vi "handle name deletion.vi"(2 "error in (no error)":errorcluster, 3 "String":string, 4 "VISA resource name":refnum<visa-resource-name>) -> (0 "error out":errorcluster, 1 "VISA resource name out":refnum<visa-resource-name>)   [LabVIEW 2018]
uses:
  <instrlib>/Tektronix AWG 5000 7000 Series/Tektronix AWG 5000 7000 Series.lvlib
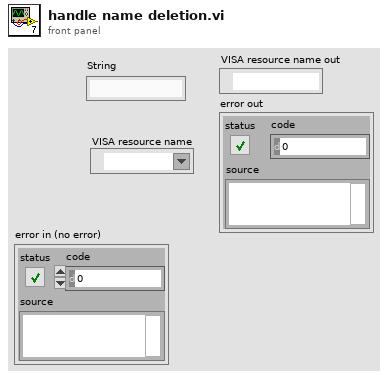
[diagram p1: front panel]
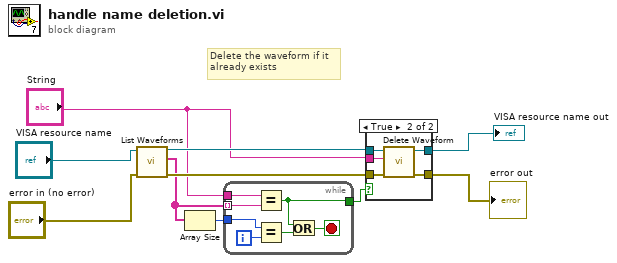
[diagram p0: block diagram]
diagram:
  # "Delete the waveform if it\nalready exists"
  n1 = call <instrlib>:"List Waveforms.vi"("error in (no error)"="error in (no error)", "VISA resource name"="VISA resource name") -> ("error out"=w9:errorcluster, "Waveform List"=w6:string[], "VISA resource name out"=w10:refnum<visa-resource-name>)  [unwired: 7 in]
  n2 = Array Size(array=w6) -> (size(s)=w7:i32)
  n3 = while {
    tunnel: [w15] -> w8
    tunnel: w7 -> [w13]
    tunnel: "String" -> [w12]
    tunnel: w6 -> [w11] mode=indexing
    i -> [w17]
    stop <- w14 stop-if-true
    n4 = Equal?(x=w12, y=w11) -> (x = y?=w15:bool)
    n5 = Equal?(x=w13, y=w17) -> (x = y?=w16:bool)
    n6 = Or(x=w15, y=w16) -> (x .or. y?=w14:bool)
  }
  n7 = case shown="True" w8 {
    tunnel: w10 -> [w19 w24]
    tunnel: [w19 w23] -> w4
    tunnel: w9 -> [w18 w22]
    tunnel: [w18 w21] -> w3
    tunnel: "String" -> [_ w20]
    frame False {
    }
    frame True {
      n8 = call <instrlib>:"Delete Waveform.vi"("error in (no error)"=w22, "Waveform Name"=w20, "VISA resource name"=w24) -> ("error out"=w21:errorcluster, "VISA resource name out"=w23:refnum<visa-resource-name>)  [unwired: 7 in]
    }
  }
  "VISA resource name out" <- w4
  "error out" <- w3
